vi "SS Class Telescope Gen Channel.vi"() -> (3 "Channel List":refnum<class "HK Item.lvclass">[](array[class]))   [LabVIEW 2024, in "Subsystem Telescope.lvclass"]
uses:
  Subsystem Telescope.lvclass
  hk-channel-class/hk-channel-class/HK Item/HK Item.lvclass
  hk-channel-class/hk-channel-class/HK Item/HK Channel Units and Setup.ctl
  hk-channel-class/hk-channel-class/HK Item/HK Channel enum Data Type.ctl
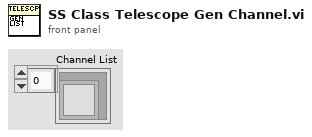
[diagram p1: front panel]
types:
  T1 = typedef "HK Item.lvclass/HK Channel Units and Setup.ctl" = cluster{"Unit Type":string, "Units":string, "Configuration":string, "Digits":i32, "Data Type":T2, "Exponential?":bool, "Source":string}
  T2 = typedef "HK Item.lvclass/HK Channel enum Data Type.ctl" = enum16{"Floating Point", "Integer", "Enum", "String", "Waveform", "File"}
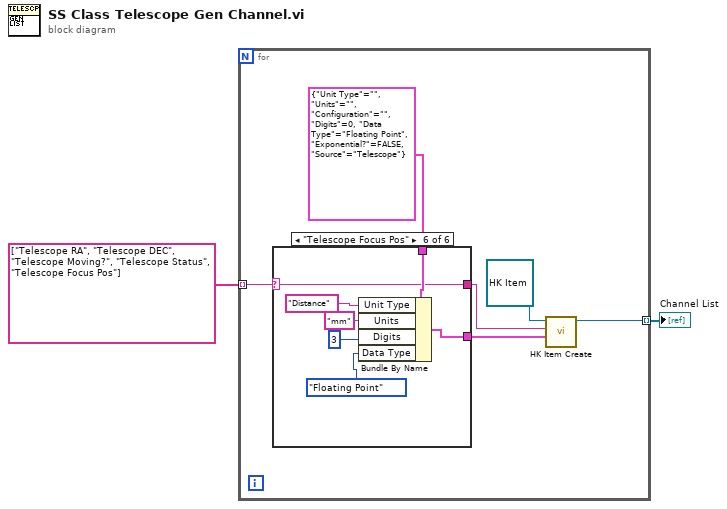
[diagram p0: block diagram]
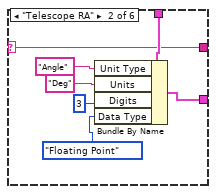
[diagram p3: hidden frame]
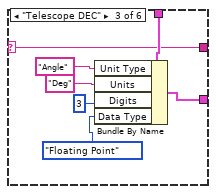
[diagram p4: hidden frame]
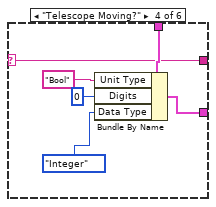
[diagram p5: hidden frame]
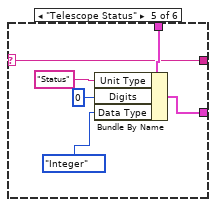
[diagram p6: hidden frame]
diagram:
  n1 = for {
    tunnel: string[] ["Telescope RA", "Telescope DEC", "Telescope Moving?", "Telescope Status", "Telescope Focus Pos"] -> [w8] mode=indexing
    tunnel: [w4] -> w1 mode=indexing
    n2 = case shown="\"Telescope Focus Pos\"" w8 {
      selector: w8 -> [w10 w11 w18 w25 w31 w38]
      tunnel: T1 {"Unit Type"="", "Units"="", "Configuration"="", "Digits"=0, "Data Type"=enum."Floating Point", "Exponential?"=FALSE, "Source"="Telescope"} ("Channel Setup") -> [w9 w17 w24 w30 w36 w43]
      tunnel: [w9 w12 w19 w26 w32 w39] -> w7
      tunnel: [w10 w11 w18 w25 w31 w38] -> w6
      frame "False", Default {
      }
      frame "Telescope RA" {
        n3 = Bundle By Name(cluster=w17, "Unit Type"="Angle", "Units"="Deg", "Digits"=3, "Data Type"=HK_Channel_enum_Data_Type."Floating Point") -> (w12:T1)
      }
      frame "Telescope DEC" {
        n4 = Bundle By Name(cluster=w24, "Unit Type"="Angle", "Units"="Deg", "Digits"=3, "Data Type"=HK_Channel_enum_Data_Type."Floating Point") -> (w19:T1)
      }
      frame "Telescope Moving?" {
        n5 = Bundle By Name(cluster=w30, "Unit Type"="Bool", "Digits"=0, "Data Type"=HK_Channel_enum_Data_Type."Integer") -> (w26:T1)
      }
      frame "Telescope Status" {
        n6 = Bundle By Name(cluster=w36, "Unit Type"="Status", "Digits"=0, "Data Type"=HK_Channel_enum_Data_Type."Integer") -> (w32:T1)
      }
      frame "Telescope Focus Pos" {
        n7 = Bundle By Name(cluster=w43, "Unit Type"="Distance", "Units"="mm", "Digits"=3, "Data Type"=HK_Channel_enum_Data_Type."Floating Point") -> (w39:T1)
      }
    }
    n8 = call-dynamic "HK Item Create.vi"("Channel Setup"=w7, "Name"=w6, "HK Item in"=refnum<class "HK Item.lvclass"> refnum) -> ("HK Item out"=w4:refnum<class "HK Item.lvclass">)  [unwired: 7 in, 1 out]
  }
  "Channel List" <- w1
